vi "RunTest.vi"(8 "error in (no error)":errorcluster, 11 "Theory in":refnum<class "Theory.lvclass">) -> (0 "error out":errorcluster, 3 "Theory out":refnum<class "Theory.lvclass">)   [LabVIEW 2019, in "TestCase.lvlib" / "Theory.lvclass"]
doc: "Override to run the test and assert its state."
uses:
  Theory.lvclass
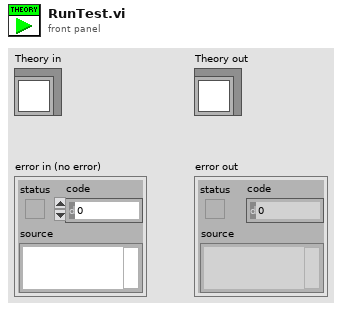
[diagram p1: front panel]
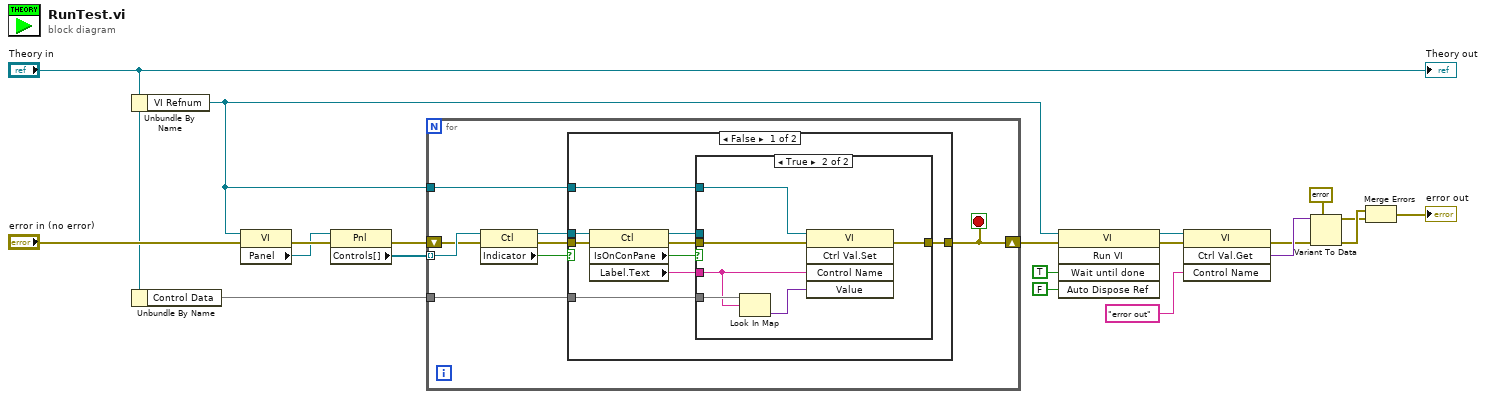
[diagram p0: block diagram]
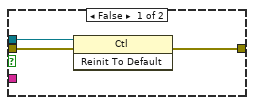
[diagram p2: hidden frame]
diagram:
  n1 = Unbundle By Name("Theory in") -> ("VI Refnum"=w1:refnum<vi>)
  n2 = Unbundle By Name("Theory in") -> ("Control Data"=w19:map{string, variant})
  n3 = property class="VI"(reference=w1, error in="error in (no error)") -> (error out=w18:errorcluster, "Panel"=w16:refnum<vi>)  [unwired: 1 out]
  n4 = property class="Pnl"(reference=w16, error in=w18) -> (error out=w17:errorcluster, "Controls[]"=w15:refnum<vi>[])  [unwired: 1 out]
  n5 = for {
    tunnel: w1 -> [w27]
    shift-right: [w26] -> w4
    shift-left: w17 -> [w24]
    tunnel: w19 -> [w28]
    tunnel: w15 -> [w25] mode=indexing
    stop <- w26 stop-if-true
    n6 = property class="Ctl"(reference=w25, error in=w24) -> (reference out=w23:refnum<vi>, error out=w22:errorcluster, "Indicator"=w21:bool)
    n7 = case shown="False" w21 {
      tunnel: w28 -> [w35 _]
      tunnel: w27 -> [w32 _]
      tunnel: [w31 w47] -> w26
      tunnel: w23 -> [w30 _]
      tunnel: w22 -> [w29 w47]
      frame False {
        n8 = property class="Ctl"(reference=w30, error in=w29) -> (reference out=w33:refnum<vi>, error out=w36:errorcluster, "IsOnConPane"=w37:bool, "Label.Text"=w34:string)
        n9 = case shown="True" w37 {
          tunnel: [w39 w41] -> w31
          tunnel: w36 -> [w40 w45]
          tunnel: w35 -> [_ w46]
          tunnel: w34 -> [_ w43]
          tunnel: w33 -> [w38 _]
          tunnel: w32 -> [_ w44]
          frame False {
            n10 = invoke class="Ctl" method="Reinit To Default"(reference=w38, error in=w40) -> (error out=w39:errorcluster)  [unwired: 1 in, 2 out]
          }
          frame True {
            n11 = Look In Map(map=w46, key=w43) -> (value=w42:variant)  [unwired: 1 in, 1 out]
            n12 = invoke class="VI" method="Ctrl Val.Set"(reference=w44, error in=w45, "Control Name"=w43, "Value"=w42) -> (error out=w41:errorcluster)  [unwired: 1 in, 4 out]
          }
        }
      }
      frame True {
      }
    }
  }
  n13 = invoke class="VI" method="Run VI"(reference=w1, error in=w4, "Wait until done"=TRUE ("Wait Until Done"), "Auto Dispose Ref"=FALSE ("Auto Dispose Reference")) -> (reference out=w11:refnum<vi>, error out=w10:errorcluster)  [unwired: 1 in, 3 out]
  n14 = invoke class="VI" method="Ctrl Val.Get"(reference=w11, error in=w10, "Control Name"="error out") -> (error out=w5:errorcluster, "Get Control Value Variant"=w8:variant)  [unwired: 1 in, 2 out]
  n15 = Variant To Data(error in=w5, type=errorcluster {"status"=FALSE, "code"=0, "source"=""}, Variant=w8) -> (data=w6:errorcluster, error out=w9:errorcluster)
  n16 = Merge Errors(w9, w6) -> (→"error out":errorcluster)
  "Theory out" <- "Theory in"
